vi "Acquisition Message Loop.vi"(8 "error in (no error)":errorcluster, 9 "Data Queue":refnum<queue>, 10 "Data Notifier":refnum<notifier>, 11 "Message Queues":T1) -> (0 "error out":errorcluster)   [LabVIEW 2017, in "Acquisition.lvlib"]
doc: "Message loop for handling messages pertaining to the acquisition of data from the hardware."
uses:
  Acquisition.lvlib
  support/Message Queue/All Message Queues.ctl
  support/Message Queue/Message Cluster.ctl
  Hardware Configuration.ctl
  Acquisition State.ctl
  support/Message Queue/Enqueue Message (Single).vi
  <vilib>/Utility/error.llb/Error Cluster From Error Code.vi
  <vilib>/ErrorRing/Error Ring.xnode
  support/Message Queue/Message Queue.lvlib
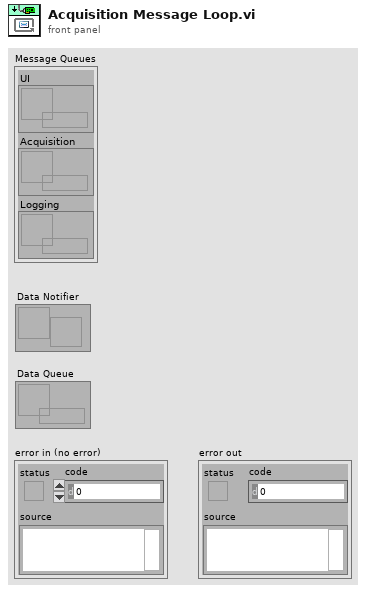
[diagram p1: front panel]
types:
  T1 = typedef "Message Queue.lvlib/All Message Queues.ctl" = cluster{"UI":refnum<queue>, "Acquisition":refnum<queue>, "Logging":refnum<queue>}
  T2 = typedef "Acquisition.lvlib/Hardware Configuration.ctl" = cluster{"DAQmx Channel":string, "Sample Rate":dbl, "DAQmx Task":refnum<k21>, "ResetInterp":bool, "GainConstants":dbl[], "FilterCoefficients":dbl[][], "ChannelNames":string[], "ActiveChannels":i32[], "Display Rate":i32, "ResponseExtension":bool}
  T3 = typedef "Acquisition.lvlib/Acquisition State.ctl" = enum16{"Idle", "Acquiring"}
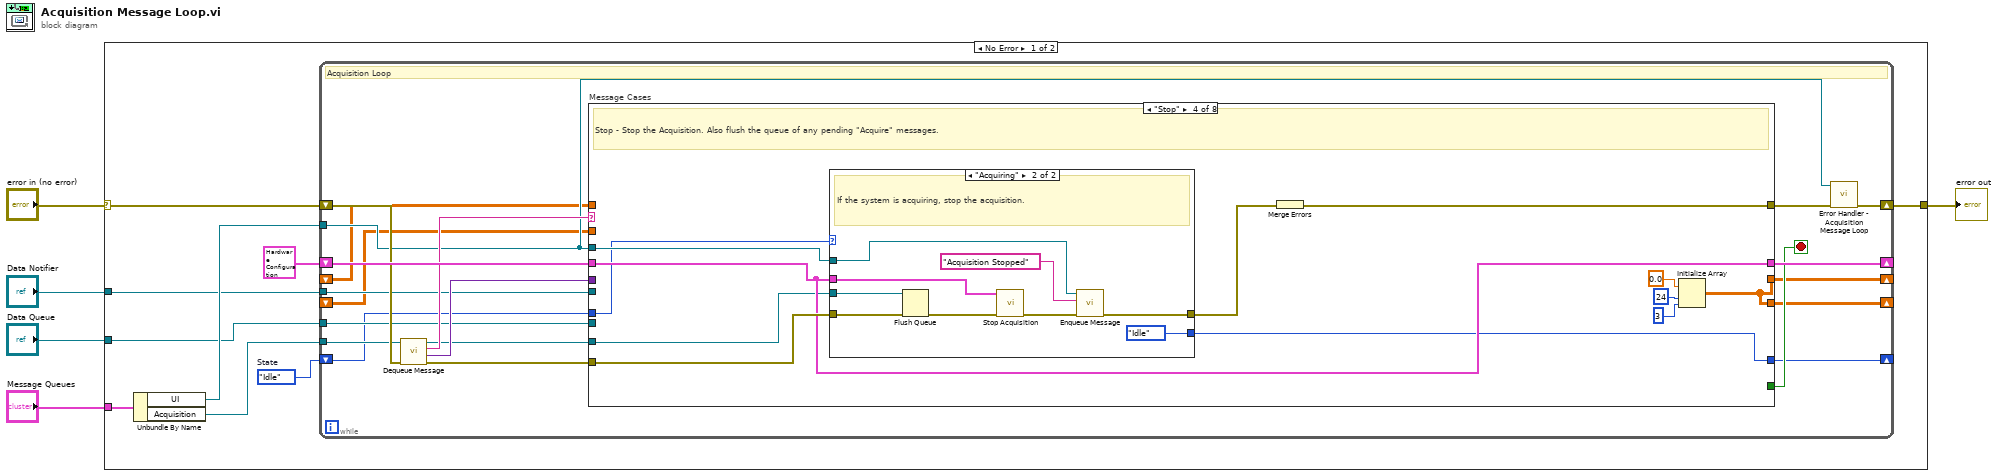
[diagram p0: block diagram]
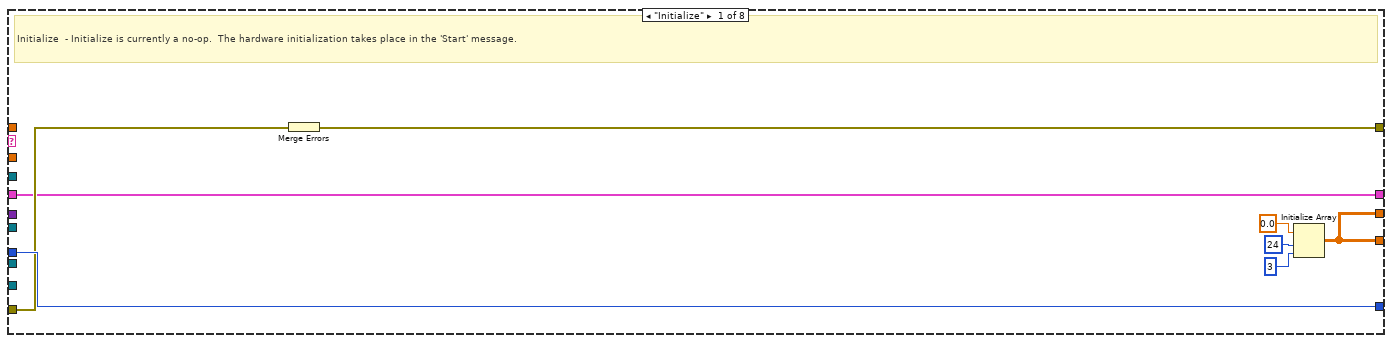
[diagram p2: hidden frame]
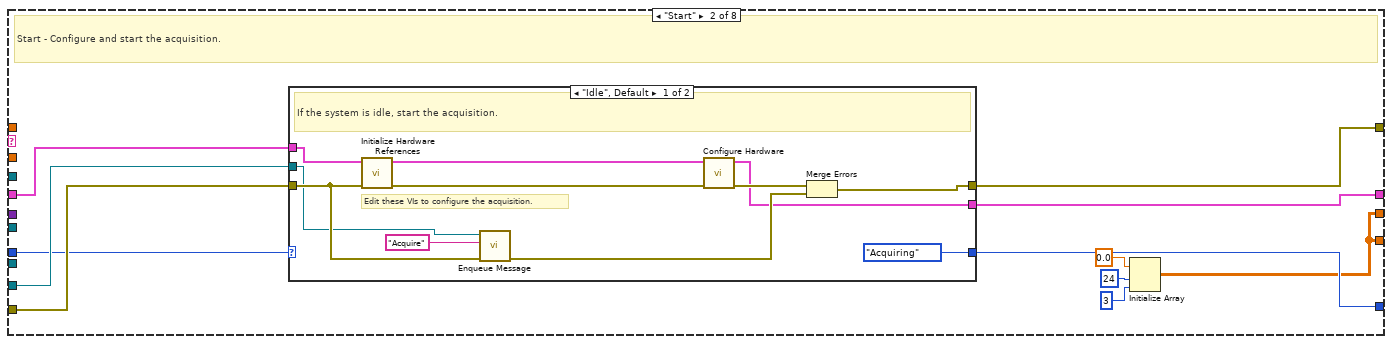
[diagram p3: hidden frame]
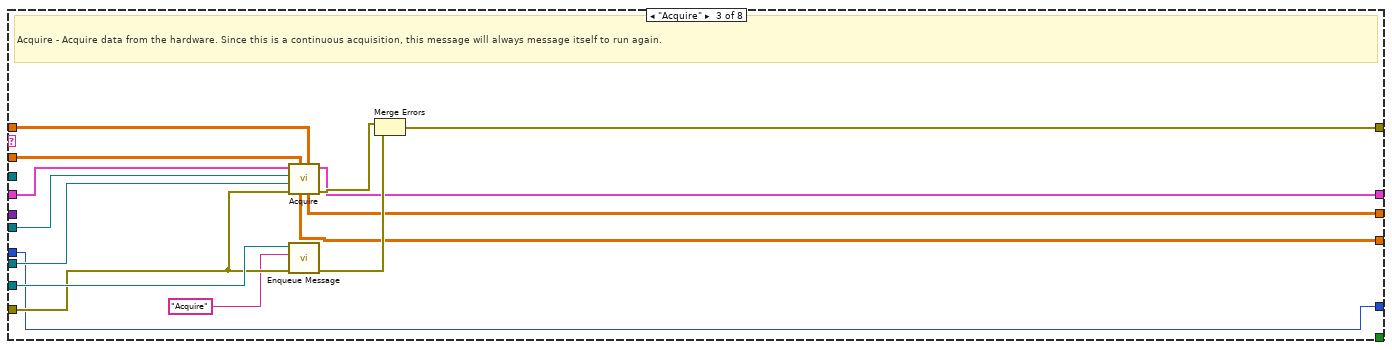
[diagram p5: hidden frame]
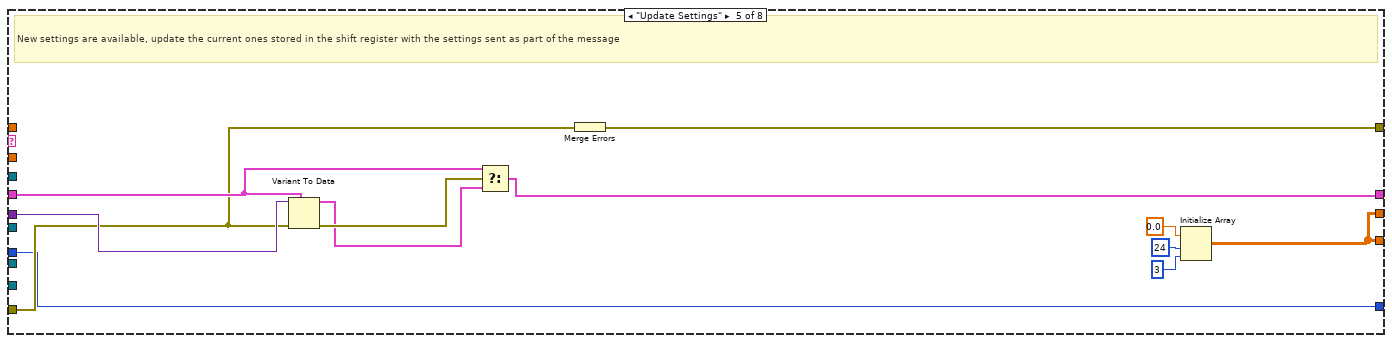
[diagram p7: hidden frame]
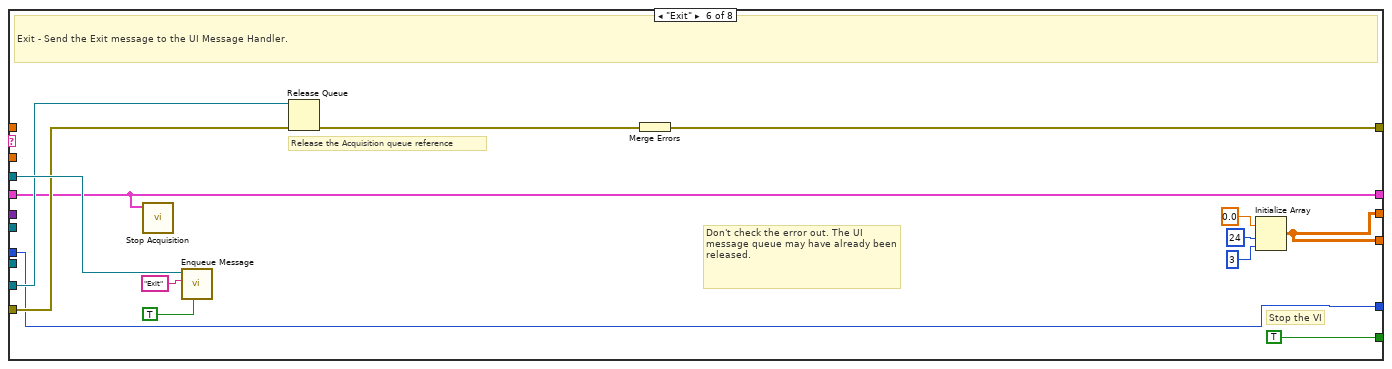
[diagram p8: hidden frame]
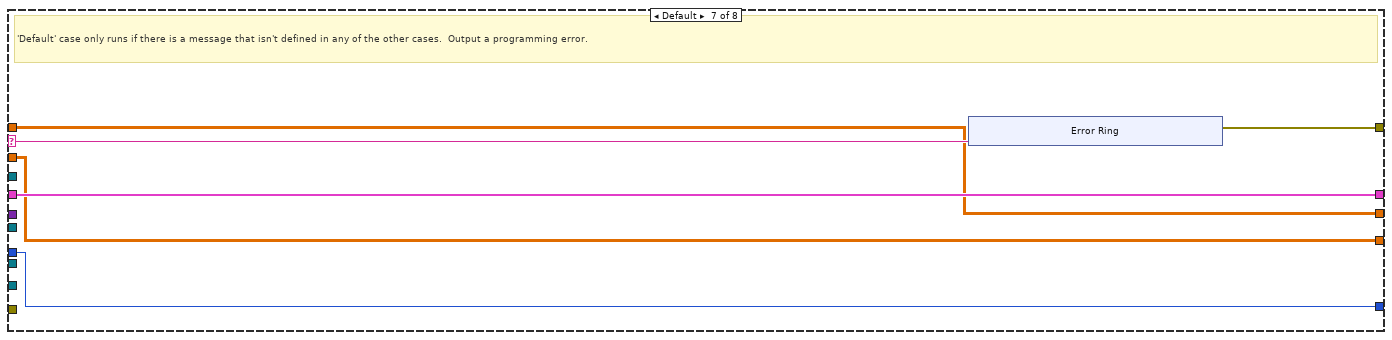
[diagram p9: hidden frame]
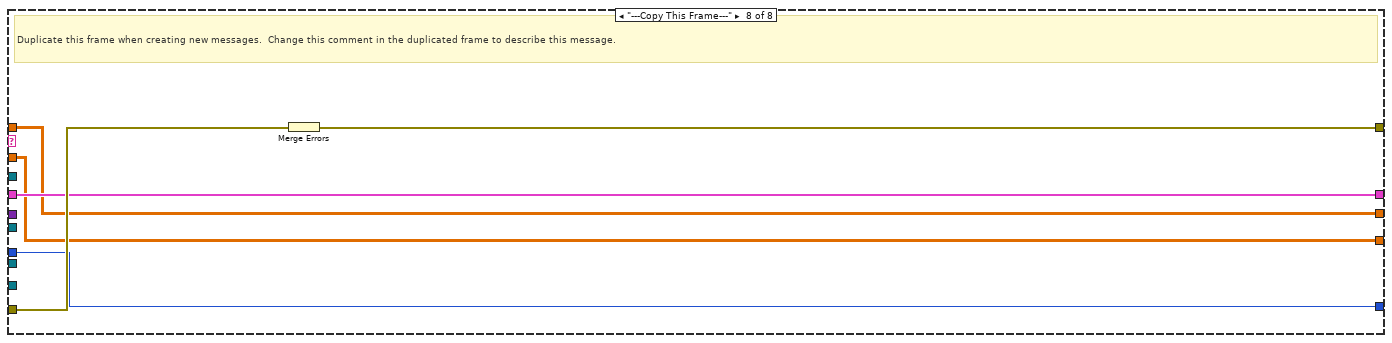
[diagram p10: hidden frame]
diagram:
  n1 = case shown="No Error" "error in (no error)" {
    selector: "error in (no error)" -> [w10 w151]
    tunnel: "Message Queues" -> [w14 _]
    tunnel: [w12 w151] -> w4
    tunnel: "Data Notifier" -> [w8 _]
    tunnel: "Data Queue" -> [w7 _]
    frame No Error {
      w6 = Acquisition_State."Idle"  # State
      n2 = Unbundle By Name(w14) -> ("UI"=w9:refnum<queue>, "Acquisition"=w13:refnum<queue>)
      n3 = while {
        tunnel: w13 -> [w26]
        shift-right: [w33] -> _
        shift-left: T2 {"DAQmx Channel"="", "Sample Rate"=0.0, "DAQmx Task"="", "ResetInterp"=FALSE, "GainConstants"=[2.0, 10.0, 1.0, 0.1, 0.01, 0.001], "FilterCoefficients"=[], "ChannelNames"=[], "ActiveChannels"=[], "Display Rate"=1000, "ResponseExtension"=TRUE} ("Data Cluster") -> [w34]
        shift-right: [w22] -> w12
        shift-left: w10 -> [w31]
        tunnel: w9 -> [w21]
        tunnel: w8 -> [w25]
        tunnel: w7 -> [w24]
        shift-right: [w19] -> _
        shift-left: w6 -> [w20]
        shift-right: [w18] -> _
        shift-left: _ -> [w16]
        shift-right: [w17] -> _
        shift-left: _ -> [w15]
        stop <- w32 stop-if-true
        # "Acquisition Loop"
        n4 = call "Dequeue Message.vi"("error in (no error)"=w31, "Message Queue"=w26) -> ("error out"=w30:errorcluster, "Message Data"=w28:variant, "Message"=w29:string, "dup Message Queue"=w27:refnum<queue>)  [unwired: 6 in]
        n5 = case "Message Cases" shown="\"Stop\"" w29 {
          selector: w29 -> [_ _ _ _ _ _ w136 _]
          tunnel: w27 -> [_ w50 w80 w91 _ w124 _ _]
          tunnel: w30 -> [w40 w51 w79 w93 w111 w128 _ w150]
          tunnel: [w42 w53 w82 w94 w117 w130 w135 w148] -> w23
          tunnel: w34 -> [w39 w52 w76 w92 w113 w123 w137 w149]
          tunnel: [w39 w49 w77 w92 w112 w123 w137 w149] -> w33
          tunnel: [_ _ _ _ _ TRUE _ _] -> w32
          tunnel: w28 -> [_ _ _ _ w116 _ _ _]
          tunnel: w21 -> [_ _ _ w90 _ w129 _ _]
          tunnel: w25 -> [_ _ w74 _ _ _ _ _]
          tunnel: w24 -> [_ _ w73 _ _ _ _ _]
          tunnel: w20 -> [w41 w48 w72 w89 w110 w122 w134 w147]
          tunnel: [w41 w47 w72 w88 w110 w122 w134 w147] -> w19
          tunnel: [w38 w43 w71 w83 w106 w118 w133 w146] -> w18
          tunnel: [w38 w43 w70 w83 w106 w118 w132 w145] -> w17
          tunnel: w16 -> [_ _ w69 _ _ _ w133 w146]
          tunnel: w15 -> [_ _ w68 _ _ _ w132 w145]
          frame "Initialize" {
            # "Initialize  - Initialize is currently a no-op.  The hardware initialization takes place in the 'Start' message."
            n6 = Merge Errors(w40) -> (w42:errorcluster)
            n7 = Initialize Array(0.0 ("element"), 24 ("dimension size"), 3 ("dimension size")) -> (w38:dbl[][])
          }
          frame "Start" {
            # "Start - Configure and start the acquisition."
            n8 = case shown="\"Idle\", Default" w48 {
              selector: w48 -> [_ w65]
              tunnel: [w64 w67] -> w53
              tunnel: w52 -> [w63 w66]
              tunnel: w51 -> [w62 w67]
              tunnel: w50 -> [w60 _]
              tunnel: [w56 w66] -> w49
              tunnel: [Acquisition_State."Acquiring" ("State") w65] -> w47
              frame "Idle", Default {
                # "Edit these VIs to configure the acquisition."
                # "If the system is idle, start the acquisition."
                n9 = call "Initialize Hardware References.vi"("error in (no error)"=w62, "Hardware Resources in"=w63) -> ("error out"=w59:errorcluster, "Hardware Resources out"=w57:T2)  [unwired: 8 in]
                n10 = call-poly "Enqueue Message.vi"("error in (no error)"=w62, "Message"="Acquire", "Message Queue"=w60) -> ("error out"=w61:errorcluster)  [unwired: 7 in, 1 out]
                n11 = call "Configure Hardware.vi"("error in (no error)"=w59, "Hardware Resources in"=w57) -> ("error out"=w58:errorcluster, "Hardware Resources out"=w56:T2)  [unwired: 8 in]
                n12 = Merge Errors(w58, w61) -> (w64:errorcluster)
              }
              frame "Acquiring" {
                # "The system is already acquiring. Ignore the \"Start\" message."
              }
            }
            n13 = Initialize Array(0.0 ("element"), 24 ("dimension size"), 3 ("dimension size")) -> (w43:dbl[][])
          }
          frame "Acquire" {
            # "Acquire - Acquire data from the hardware. Since this is a continuous acquisition, this message will always message itself to run again."
            n14 = call "Acquire.vi"("Initial Y Conditions"=w69, "Initial X Conditions"=w68, "error in (no error)"=w79, "Data Queue"=w73, "Data Notifier"=w74, "Hardware Resources in"=w76) -> ("error out"=w78:errorcluster, "Hardware Resources out"=w77:T2, "Final Y Conditions"=w71:dbl[][], "Final X Conditions"=w70:dbl[][])  [unwired: 2 in]
            n15 = call-poly "Enqueue Message.vi"("error in (no error)"=w79, "Message"="Acquire", "Message Queue"=w80) -> ("error out"=w81:errorcluster)  [unwired: 7 in, 1 out]
            n16 = Merge Errors(w78, w81) -> (w82:errorcluster)
          }
          frame "Stop" {
            # "Stop - Stop the Acquisition. Also flush the queue of any pending \"Acquire\" messages."
            n17 = case shown="\"Acquiring\"" w89 {
              selector: w89 -> [w96 _]
              tunnel: w93 -> [w95 w105]
              tunnel: w92 -> [_ w104]
              tunnel: w91 -> [_ w102]
              tunnel: w90 -> [_ w101]
              tunnel: [w96 Acquisition_State."Idle" ("State")] -> w88
              tunnel: [w95 w99] -> w87
              frame "Idle", Default {
                # "The system is already idle. Ignore the \"Stop\" message."
              }
              frame "Acquiring" {
                # "If the system is acquiring, stop the acquisition."
                n18 = Flush Queue(queue=w102, error in (no error)=w105) -> (error out=w103:errorcluster)  [unwired: 2 out]
                n19 = call "Stop Acquisition.vi"("error in (no error)"=w103, "Hardware Resources in"=w104) -> ("error out"=w100:errorcluster)  [unwired: 9 in]
                n20 = call-poly "Enqueue Message.vi"("error in (no error)"=w100, "Message"="Acquisition Stopped", "Message Queue"=w101) -> ("error out"=w99:errorcluster)  [unwired: 7 in, 1 out]
              }
            }
            n21 = Merge Errors(w87) -> (w94:errorcluster)
            n22 = Initialize Array(0.0 ("element"), 24 ("dimension size"), 3 ("dimension size")) -> (w83:dbl[][])
          }
          frame "Update Settings" {
            # "New settings are available, update the current ones stored in the shift register with the settings sent as part of the message"
            n23 = Variant To Data(error in=w111, type=w113, Variant=w116) -> (data=w114:T2, error out=w115:errorcluster)
            n24 = Select(t=w113, s=w115, f=w114) -> (s? t:f=w112:T2)
            n25 = Merge Errors(w111) -> (w117:errorcluster)
            n26 = Initialize Array(0.0 ("element"), 24 ("dimension size"), 3 ("dimension size")) -> (w106:dbl[][])
          }
          frame "Exit" {
            # "Don't check the error out. The UI message queue may have already been released."
            # "Release the Acquisition queue reference"
            # "Stop the VI"
            # "Exit - Send the Exit message to the UI Message Handler."
            n27 = call "Stop Acquisition.vi"("Hardware Resources in"=w123) -> ()  [unwired: 10 in, 1 out]
            n28 = call-poly "Enqueue Message.vi"("Priority Message? (F)"=TRUE, "Message"="Exit", "Message Queue"=w129) -> ()  [unwired: 7 in, 2 out]
            n29 = Release Queue(queue=w124, error in (no error)=w128) -> (error out=w125:errorcluster)  [unwired: 1 in, 2 out]
            n30 = Merge Errors(w125) -> (w130:errorcluster)
            n31 = Initialize Array(0.0 ("element"), 24 ("dimension size"), 3 ("dimension size")) -> (w118:dbl[][])
          }
          frame Default {
            # "'Default' case only runs if there is a message that isn't defined in any of the other cases.  Output a programming error."
            n32 = xnode "Error Ring"("parameter 0"=w136) -> ("error out"=w135:errorcluster)
          }
          frame "---Copy This Frame---" {
            # "Duplicate this frame when creating new messages.  Change this comment in the duplicated frame to describe this message."
            n33 = Merge Errors(w150) -> (w148:errorcluster)
          }
        }
        n34 = call "Error Handler - Acquisition Message Loop.vi"("error in (no error)"=w23, "Message Queue"=w21) -> ("dup error in"=w22:errorcluster)  [unwired: 8 in, 1 out]
      }
    }
    frame Error {
    }
  }
  "error out" <- w4
